vi "Update Zones Booleans.vi"(8 "error in (no error)":errorcluster, 11 "Model Data in":T1={"Position"=0.0, "Settings"={"Length [m]"=20.0, "Dose Zone Start"=8.0, "Dose Zone  End"=12.0, "Barrel Volume [l]"=100.0, "Dosing level [l]"=90.0}, "Pump State"=FALSE, "Fluid Flow"=0.0, "Inpute Zone"=FALSE, "Dosing Zone"=FALSE, "Output Zone"=FALSE, "UI Refs"={"DOSING"=refnum, "INPUT"=refnum, "OUTPUT"=refnum, "Pump"=refnum, "Fluid Level [l]"=refnum, "Flow [l/s]"=refnum, "Production line"=refnum, "SPILL"=refnum, "LOW LEVEL"=refnum, "Barrel Number"=refnum}, "Fluid Level"=0.0, "Barrel Number"=0, "Spill Alarm"=FALSE, "Level Alarm"=FALSE, "millisecond timer value"=0, "Start simulation"=FALSE}) -> (0 "error out":errorcluster, 2 "Zone change?":bool, 3 "Model Data out":T1={"Position"=0.0, "Settings"={"Length [m]"=20.0, "Dose Zone Start"=8.0, "Dose Zone  End"=12.0, "Barrel Volume [l]"=100.0, "Dosing level [l]"=90.0}, "Pump State"=FALSE, "Fluid Flow"=0.0, "Inpute Zone"=FALSE, "Dosing Zone"=FALSE, "Output Zone"=FALSE, "UI Refs"={"DOSING"=refnum, "INPUT"=refnum, "OUTPUT"=refnum, "Pump"=refnum, "Fluid Level [l]"=refnum, "Flow [l/s]"=refnum, "Production line"=refnum, "SPILL"=refnum, "LOW LEVEL"=refnum, "Barrel Number"=refnum}, "Fluid Level"=0.0, "Barrel Number"=0, "Spill Alarm"=FALSE, "Level Alarm"=FALSE, "millisecond timer value"=0, "Start simulation"=FALSE})   [LabVIEW 2016, in "Model.lvlib"]
uses:
  Model.lvlib
  TypeDefs/Model Data.ctl
  TypeDefs/PL Settings.ctl
  TypeDefs/PL UI Refs.ctl
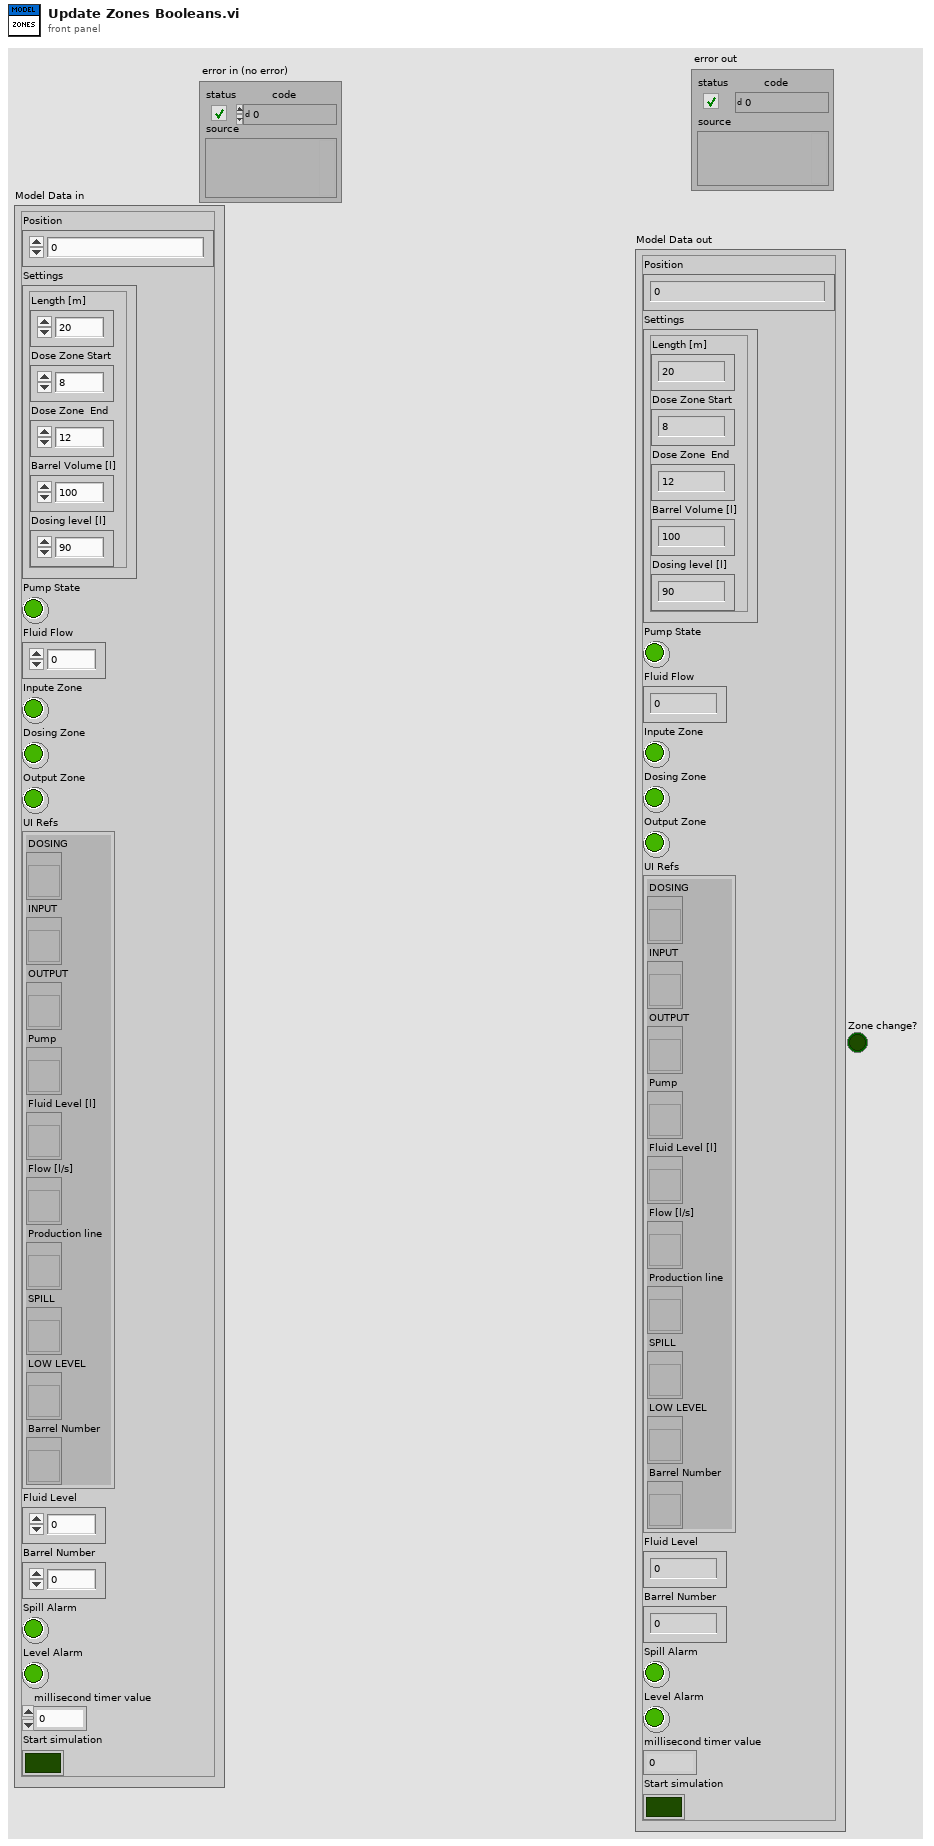
[diagram p1: front panel]
types:
  T1 = typedef "Model.lvlib/Model Data.ctl" = cluster{"Position":dbl, "Settings":T2, "Pump State":bool, "Fluid Flow":dbl, "Inpute Zone":bool, "Dosing Zone":bool, "Output Zone":bool, "UI Refs":T3, "Fluid Level":dbl, "Barrel Number":i32, "Spill Alarm":bool, "Level Alarm":bool, "millisecond timer value":u32, "Start simulation":bool}
  T2 = typedef "Model.lvlib/PL Settings.ctl" = cluster{"Length [m]":dbl, "Dose Zone Start":dbl, "Dose Zone  End":dbl, "Barrel Volume [l]":dbl, "Dosing level [l]":dbl}
  T3 = typedef "Model.lvlib/PL UI Refs.ctl" = cluster{"DOSING":refnum<vi>, "INPUT":refnum<vi>, "OUTPUT":refnum<vi>, "Pump":refnum<vi>, "Fluid Level [l]":refnum<vi>, "Flow [l/s]":refnum<vi>, "Production line":refnum<vi>, "SPILL":refnum<vi>, "LOW LEVEL":refnum<vi>, "Barrel Number":refnum<vi>}
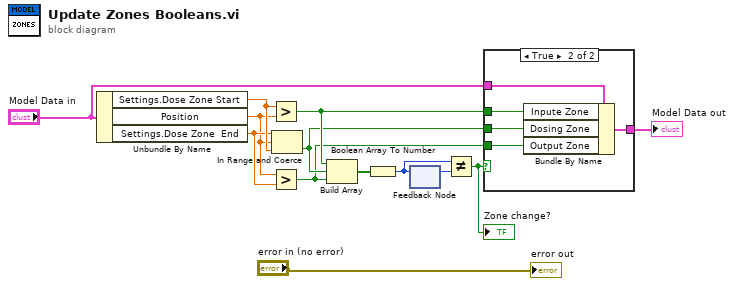
[diagram p0: block diagram]
diagram:
  n1 = Unbundle By Name("Model Data in") -> ("Settings.Dose Zone Start"=w13:dbl, "Position"=w11:dbl, "Settings.Dose Zone  End"=w12:dbl)
  n2 = Greater?(x=w13, y=w11) -> (0:w5:bool)
  n3 = Greater?(x=w11, y=w12) -> (0:w3:bool)
  n4 = In Range and Coerce(upper limit=w12, x=w11, lower limit=w13) -> (In Range?=w4:bool)  [unwired: 1 out]
  n5 = Build Array(w5, w4, w3) -> (w6:bool[])
  n6 = Boolean Array To Number(Boolean array=w6) -> (number=w10:u32)
  n7 = feedback-in #1(w10) -> ()
  n8 = feedback #1() -> (w9:u32)  [unwired: 1 in]
  n9 = Not Equal?(x=w10, y=w9) -> (x != y?=w8:bool)
  "Zone change?" <- w8
  n10 = case shown="True" w8 {
    tunnel: "Model Data in" -> [w14 w19]
    tunnel: w5 -> [_ w18]
    tunnel: w4 -> [_ w17]
    tunnel: w3 -> [_ w16]
    tunnel: [w14 w15] -> w2
    frame False {
    }
    frame True {
      n11 = Bundle By Name(cluster=w19, "Inpute Zone"=w18, "Dosing Zone"=w17, "Output Zone"=w16) -> (w15:T1)
    }
  }
  "Model Data out" <- w2
  "error out" <- "error in (no error)"
